vi "ICM Connect.vi"(0 "Com Port":refnum<visa-resource-name>, 11 "error in (no error)":errorcluster) -> (4 "ICM Ref":refnum<class "Modbus Master.lvclass">, 15 "error out":errorcluster)   [LabVIEW 2024]
uses:
  <vilib>/NI/Modbus Library/API/Master/Modbus Master.lvclass
  <vilib>/NI/Modbus Library/API/Wrapper/Create Serial Master.vi
  <vilib>/NI/Modbus Library/API/Wrapper/API Main.lvlib
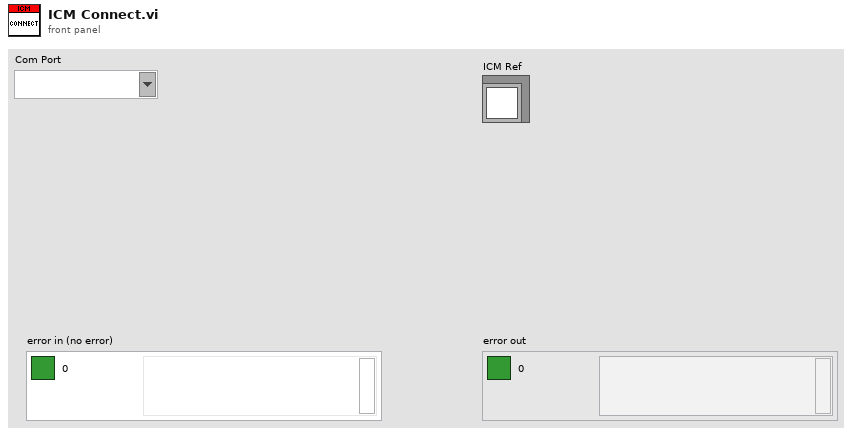
[diagram p1: front panel]
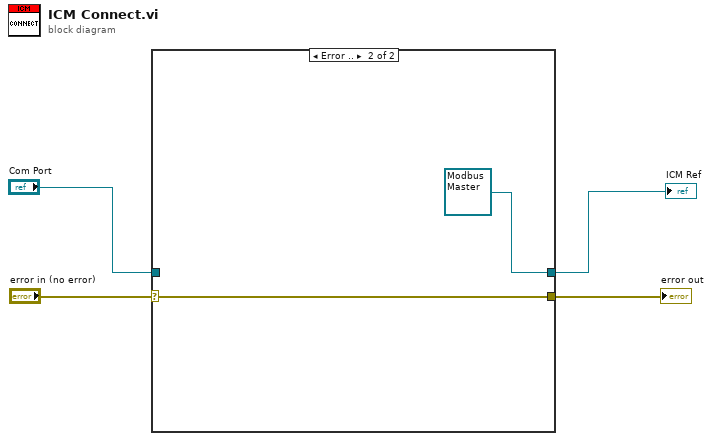
[diagram p0: block diagram]
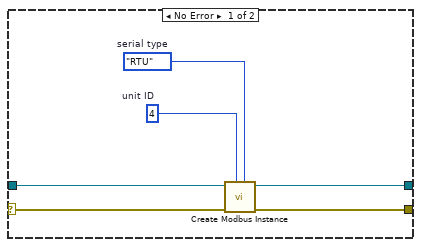
[diagram p2: hidden frame]
diagram:
  n1 = case shown="Error .." "error in (no error)" {
    selector: "error in (no error)" -> [w9 w12]
    tunnel: [w8 w12] -> w3
    tunnel: "Com Port" -> [w7 _]
    tunnel: [w5 refnum<class "Modbus Master.lvclass"> refnum ("serial master instance")] -> w1
    frame No Error {
      w6 = u8 4  # unit ID
      w10 = enum16{"RTU", "ASCII"}."RTU"  # serial type
      n2 = call-poly <vilib>:"Create Modbus Instance.vi"("serial type"=w10, "unit ID"=w6, "error in"=w9, "VISA resource name"=w7) -> ("error out"=w8:errorcluster, "serial master instance"=w5:refnum<class "Modbus Master.lvclass">)  [unwired: 6 in]
    }
    frame Error {
    }
  }
  "error out" <- w3
  "ICM Ref" <- w1
